vi "Reading Data (Sub VI).vi"(8 "error in (no error)":errorcluster, 11 "Bluetooth Network Connection in":refnum<k31>) -> (0 "error out":errorcluster, 1 "Sign bytes X":string, 2 "Sign bytes Y":string, 3 "Bluetooth Network Connection out":refnum<k31>, 4 "X data":string, 5 "Y data":string)   [LabVIEW 2012]
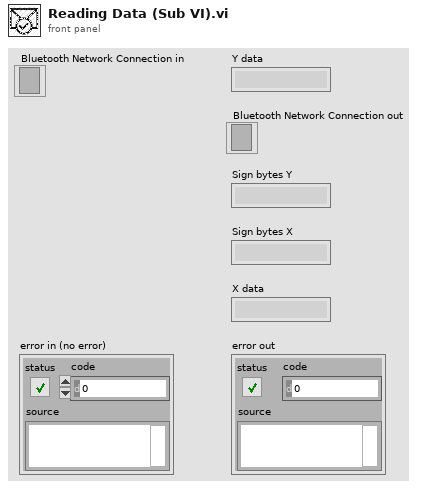
[diagram p1: front panel]
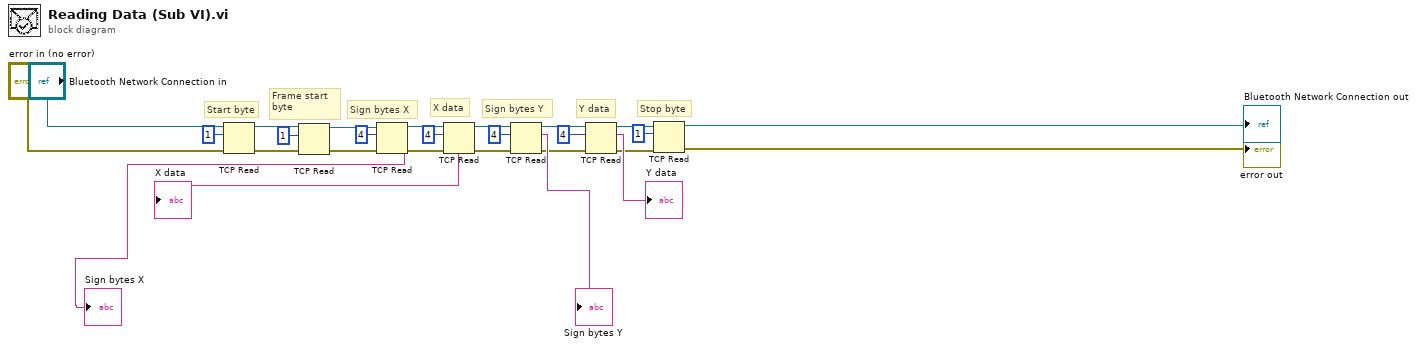
[diagram p0: block diagram]
diagram:
  # "Stop byte"
  # "Y data"
  # "Sign bytes Y"
  # "X data"
  # "Sign bytes X"
  # "Frame start byte"
  # "Start byte"
  n1 = TCP Read(connection ID="Bluetooth Network Connection in", bytes to read=u32 1 ("byte count"), error in (no error)="error in (no error)") -> (connection ID out=w2:refnum<k31>, error out=w3:errorcluster)  [unwired: 2 in, 1 out]
  n2 = TCP Read(connection ID=w2, bytes to read=u32 1 ("byte count"), error in (no error)=w3) -> (connection ID out=w11:refnum<k31>, error out=w15:errorcluster)  [unwired: 2 in, 1 out]
  n3 = TCP Read(connection ID=w11, bytes to read=u32 4 ("byte count"), error in (no error)=w15) -> (connection ID out=w12:refnum<k31>, data out=→"Sign bytes X":string, error out=w14:errorcluster)  [unwired: 2 in]
  n4 = TCP Read(connection ID=w12, bytes to read=u32 4 ("byte count"), error in (no error)=w14) -> (connection ID out=w5:refnum<k31>, data out=→"X data":string, error out=w6:errorcluster)  [unwired: 2 in]
  n5 = TCP Read(connection ID=w5, bytes to read=u32 4 ("byte count"), error in (no error)=w6) -> (connection ID out=w8:refnum<k31>, data out=→"Sign bytes Y":string, error out=w9:errorcluster)  [unwired: 2 in]
  n6 = TCP Read(connection ID=w8, bytes to read=u32 4 ("byte count"), error in (no error)=w9) -> (connection ID out=w20:refnum<k31>, data out=→"Y data":string, error out=w21:errorcluster)  [unwired: 2 in]
  n7 = TCP Read(connection ID=w20, bytes to read=u32 1 ("byte count"), error in (no error)=w21) -> (connection ID out=→"Bluetooth Network Connection out":refnum<k31>, error out=→"error out":errorcluster)  [unwired: 2 in, 1 out]
